vi "prepare.vi"(8 "error in (no error)":errorcluster, 9 "length":i32, 10 "sqlstatement pointer":i64, 11 "object in":refnum<class "SQLiteConnection.lvclass">) -> (0 "error out":errorcluster, 1 "Valid?":bool, 3 "object out":refnum<class "SQLiteConnection.lvclass">, 4 "remaining sql":i64, 5 "remaining bytes":i32)   [LabVIEW 2019, in "SQLiteConnection.lvclass"]
uses:
  SQLiteConnection.lvclass
  SQLiteConnection.lvclass/SQLiteConnection.ctl
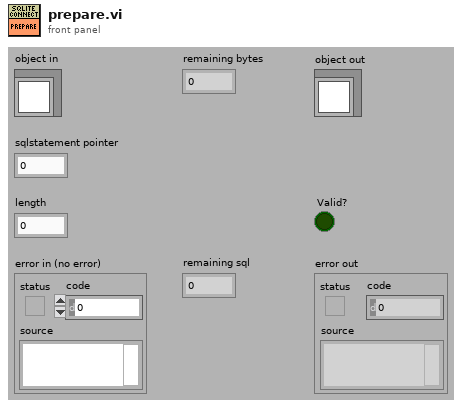
[diagram p1: front panel]
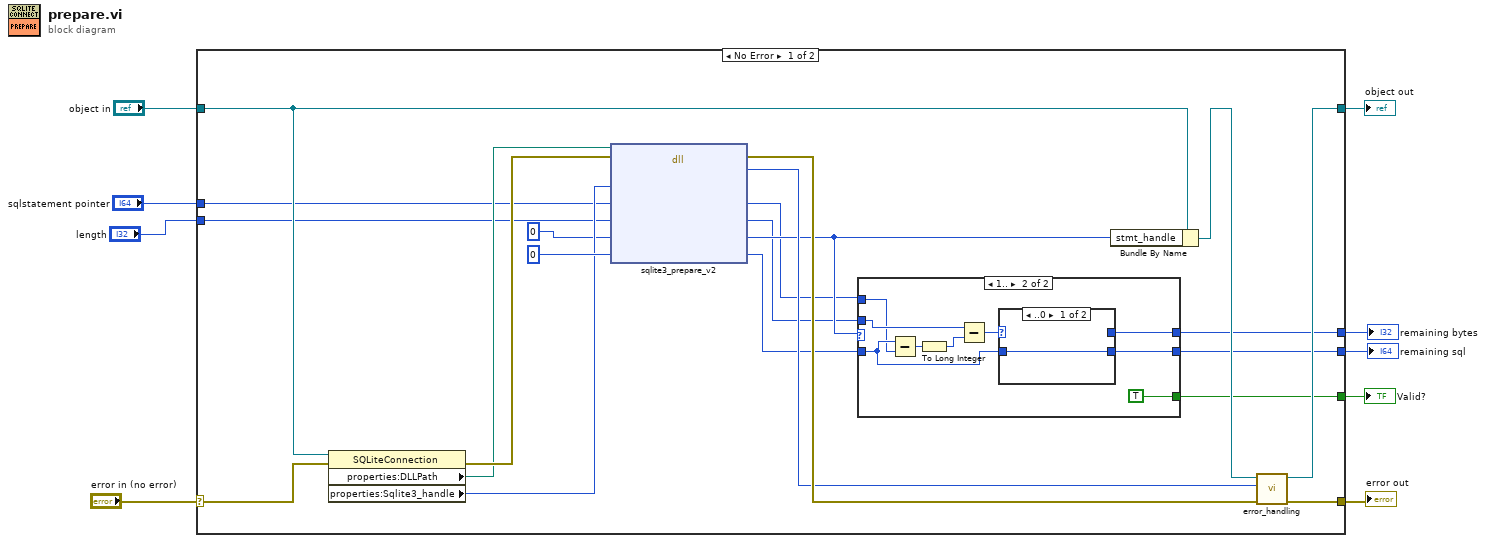
[diagram p0: block diagram]
diagram:
  n1 = case shown="No Error" "error in (no error)" {
    selector: "error in (no error)" -> [w25 w45]
    tunnel: [w29 w45] -> w8
    tunnel: [w26 w44] -> w6
    tunnel: "object in" -> [w22 w44]
    tunnel: [w15 _] -> w5
    tunnel: [w14 _] -> w4
    tunnel: [w13 _] -> w3
    tunnel: "sqlstatement pointer" -> [w11 _]
    tunnel: "length" -> [w10 _]
    frame No Error {
      n2 = property class="SQLiteConnection"(reference=w22, error in=w25) -> (error out=w23:errorcluster, "properties:DLLPath"=w21:path, "properties:Sqlite3_handle"=w20:u64)  [unwired: 1 out]
      n3 = dll-call lib="D:/Users/mcarl/Documents/LabVIEW Projects/OW-PIKO/OW-PIKO Software/sqlite3.dll" fn="sqlite3_prepare_v2"(path in=w21, error in=w23, "sqlitehandle"=w20, "sqlstatement"=w11, "length"=w10, "stmt_pointer"=u64 0, "not_used"=i64 0) -> (error out=w30:errorcluster, "return type"=w28:i32, "sqlstatement"=w18:i64, "length"=w17:i32, "stmt_pointer"=w19:u64, "not_used"=w16:i64)  [unwired: 2 in, 1 out]
      n4 = case shown="1.." w19 {
        tunnel: w16 -> [w31 w38]
        tunnel: [_ TRUE] -> w15
        tunnel: w17 -> [_ w40]
        tunnel: w18 -> [_ w37]
        tunnel: [_ w34] -> w14
        tunnel: [w31 w33] -> w13
        frame ..0 {
        }
        frame 1.. {
          n5 = Subtract(x=w38, y=w37) -> (x-y=w39:i64)
          n6 = To Long Integer(number=w39) -> (32bit integer=w32:i32)
          n7 = Subtract(x=w40, y=w32) -> (x-y=w36:i32)
          n8 = case shown="..0" w36 {
            selector: w36 -> [_ w43]
            tunnel: w38 -> [w41 w42]
            tunnel: [_ w43] -> w34
            tunnel: [w41 w42] -> w33
            frame ..0 {
            }
            frame 1.. {
            }
          }
        }
      }
      n9 = Bundle By Name(cluster=w22, "stmt_handle"=w19) -> (w27:refnum<class "SQLiteConnection.lvclass">)
      n10 = call "error_handling.vi"("error in (no error)"=w30, "error handle"=w28, "object in"=w27) -> ("error out"=w29:errorcluster, "object out"=w26:refnum<class "SQLiteConnection.lvclass">)  [unwired: 7 in]
    }
    frame Error {
    }
  }
  "error out" <- w8
  "object out" <- w6
  "Valid?" <- w5
  "remaining bytes" <- w4
  "remaining sql" <- w3
